vi "Report.PathStr.vi"(11 "FilePath In":string) -> (3 "FilePath Out":string)   [LabVIEW 2012, in "Lib_UEL.ATE.lvlib" / "Lib_Report.lvlib"]
uses:
  Lib_Report.lvlib
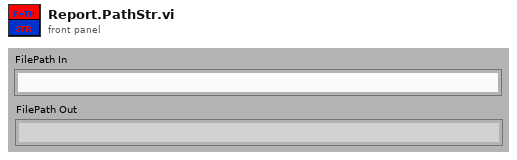
[diagram p1: front panel]
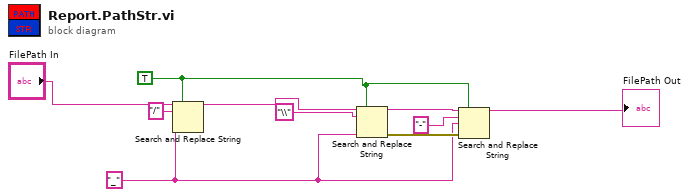
[diagram p0: block diagram]
diagram:
  w4 = TRUE ("替换全部？(F)")
  w3 = "_" ("替换字符串(\"\")")
  n1 = Search and Replace String(replace all?=w4, input string="FilePath In", search string="/" ("搜索字符串"), replace string=w3) -> (result string=w7:string)  [unwired: 4 in, 3 out]
  n2 = Search and Replace String(replace all?=w4, input string=w7, search string="\\" ("搜索字符串"), replace string=w3) -> (result string=w6:string, error out=w5:errorcluster)  [unwired: 4 in, 2 out]
  n3 = Search and Replace String(replace all?=w4, input string=w6, search string="-" ("搜索字符串"), replace string=w3, error in=w5) -> (result string=→"FilePath Out":string)  [unwired: 3 in, 3 out]
